vi "MPXsetOnOffDC.vi"(1 "Signal On":bool, 2 "MPX COM-Port":refnum<visa-resource-name>="COM5") -> (0 "MPX COM-Port dup":refnum<visa-resource-name>="COM5")   [LabVIEW 2015]
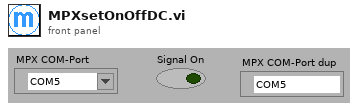
[diagram p1: front panel]
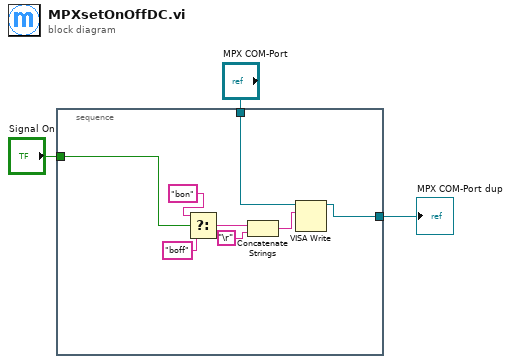
[diagram p0: block diagram]
diagram:
  n1 = stacked-sequence {
    tunnel: "MPX COM-Port" -> [w9]
    tunnel: "Signal On" -> [w8]
    tunnel: [w4] -> w1
    frame #0 {
      n2 = Select(t="bon", s=w8, f="boff") -> (s? t:f=w7:string)
      n3 = Concatenate Strings(w7, "\r") -> (w11:string)
      n4 = VISA Write(VISA resource name=w9, write buffer=w11) -> (VISA resource name out=w4:refnum<visa-resource-name>)  [unwired: 1 in, 2 out]
    }
  }
  "MPX COM-Port dup" <- w1
